vi "LED (SubVI).vi"(8 "error in (no error)":errorcluster, 11 "LED":i8) -> (0 "error out":errorcluster)   [LabVIEW 2017]
uses:
  <vilib>/myRIO/Instrument Drivers/Onboard IO/DIO/typedefs/DIO Reference.ctl
  <vilib>/myRIO/Common/Instrument Driver Framework/Utilities/typedefs/myRIO Generic Hardware Reference.ctl
  <vilib>/myRIO/Common/Instrument Driver Framework/Utilities/typedefs/Hardware Version Enum.ctl
  <vilib>/myRIO/Common/Instrument Driver Framework/Utilities/typedefs/myRIO v1.0 Reference.ctl
  <vilib>/myRIO/Common/Instrument Driver Framework/Utilities/typedefs/Generic FPGA Reference.ctl
  <vilib>/myRIO/Common/Instrument Driver Framework/myRIO v1.0/DIO/typedefs/DIO Channels List.ctl
  <vilib>/myRIO/Common/Instrument Driver Framework/myRIO v1.0/DIO/typedefs/DIO Channels Enum.ctl
  <vilib>/userdefined/High Color/nirio_resource_hc.ctl
  <vilib>/myRIO/Common/Instrument Driver Framework/Utilities/vis/Is FPGA Ref Available.vi
  <vilib>/myRIO/Common/Instrument Driver Framework/myRIO v1.0/DIO/vis/myRIO v1.1 Open DIO.vi
  <vilib>/myRIO/Instrument Drivers/Onboard IO/DIO/vis/Write.vi
  <vilib>/myRIO/Common/Instrument Driver Framework/Utilities/vis/Validate Channels.vi
  <vilib>/myRIO/Common/Instrument Driver Framework/myRIO v1.0/DIO/vis/myRIO v1.0 Reserve DIO.vi
  <vilib>/myRIO/Common/Instrument Driver Framework/myRIO v1.0/Resource Manager/vis/myRIO v1.0 Reserve Channel List.vi
  <vilib>/myRIO/Common/Instrument Driver Framework/myRIO v1.0/DIO/vis/myRIO v1.0 Build MUX Configuration DIO.vi
  <vilib>/myRIO/Common/Instrument Driver Framework/myRIO v1.0/Resource Manager/vis/myRIO v1.0 Reserve Channel.vi
  <vilib>/myRIO/Common/Instrument Driver Framework/myRIO v1.0/Resource Manager/vis/myRIO v1.0 Unreserve Channel.vi
  <vilib>/myRIO/Common/Instrument Driver Framework/myRIO v1.0/Resource Manager/vis/myRIO v1.0 Create Configuration List.vi
  <vilib>/myRIO/Common/Instrument Driver Framework/myRIO v1.0/Resource Manager/vis/myRIO v1.0 Build Mutex Name.vi
  <vilib>/Utility/VariantDataType/GetNumericInfo.vi
  <vilib>/Utility/error.llb/Error Cluster From Error Code.vi
  <vilib>/myRIO/Common/Instrument Driver Framework/myRIO v1.0/myRIO v1.1 Open.vi
  <vilib>/myRIO/Common/Instrument Driver Framework/Utilities/vis/IO Manager.vi
  <vilib>/myRIO/Common/Instrument Driver Framework/Utilities/vis/Configuration Manager.vi
  <vilib>/myRIO/Common/Instrument Driver Framework/myRIO v1.0/Resource Manager/vis/myRIO v1.0 Configure IO.vi
  <vilib>/myRIO/Common/Instrument Driver Framework/myRIO v1.0/myRIO v1.0 Close.vi
  <vilib>/myRIO/Common/Instrument Driver Framework/myRIO v1.0/DIO/vis/myRIO v1.0 Write DIO.vi
  <vilib>/myRIO/Express VI/Onboard IO/DO/DO Express VI.xnode
  <vilib>/myRIO/Instrument Drivers/Onboard IO/DIO/vis/myRIO DIO Open.xnode
  <vilib>/myRIO/Instrument Drivers/Onboard IO/DIO/DIO.lvlib
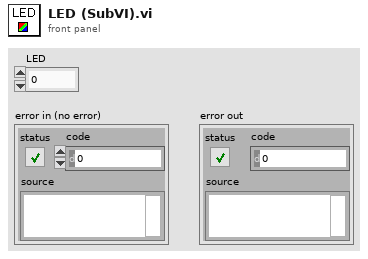
[diagram p1: front panel]
types:
  T1 = typedef "DIO.lvlib/DIO Reference.ctl" = cluster{"myRIO Reference":T2, "DIO Channels List":T6}
  T2 = typedef "myRIO Generic Hardware Reference.ctl" = cluster{"myRIO Model":T3, "myRIO Hardware Reference":T4}
  T3 = typedef "Hardware Version Enum.ctl" = enum16{"Unknown", "myRIO-1900", "myRIO-1950", "roboRIO", "NI ELVIS RIO CM"}
  T4 = typedef "myRIO v1.0 Reference.ctl" = cluster{"Generic FPGA Reference":T5, "Allow multiple opens":bool}
  T5 = typedef "Generic FPGA Reference.ctl" = refnum<k20>
  T6 = typedef "DIO Channels List.ctl" = T7[]
  T7 = typedef "DIO Channels Enum.ctl" = enum16{"Not Connected", "C/DIO0", "C/DIO1", "C/DIO2", "C/DIO3", "C/DIO4", "C/DIO5", "C/DIO6", "C/DIO7", "A/DIO0", "A/DIO1", "A/DIO2", "A/DIO3", "A/DIO4", "A/DIO5", "A/DIO6", "A/DIO7", "A/DIO8", "A/DIO9", "A/DIO10", "A/DIO11", "A/DIO12", "A/DIO13", "A/DIO14", "A/DIO15", "B/DIO0", "B/DIO1", "B/DIO2", "B/DIO3", "B/DIO4", "B/DIO5", "B/DIO6", "B/DIO7", "B/DIO8", "B/DIO9", "B/DIO10", "B/DIO11", "B/DIO12", "B/DIO13", "B/DIO14", "B/DIO15", "LED0", "LED1", "LED2", "LED3", "Button0", "DIO/DIO0", "DIO/DIO1", "DIO/DIO2", "DIO/DIO3", "DIO/DIO4", "DIO/DIO5", "DIO/DIO6", "DIO/DIO7", "DIO/DIO8", "DIO/DIO9", "SPI/CS0", "SPI/CS1", "SPI/CS2", "SPI/CS3", "LED RADIO (Green)", "LED RADIO (Red)", "LED COMM (Green)", "LED COMM (Red)", "LED MODE (Green)", "LED MODE (Red)"}
  T8 = typedef "nirio_resource_hc.ctl" = tag
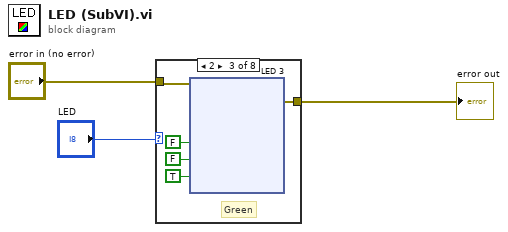
[diagram p0: block diagram]
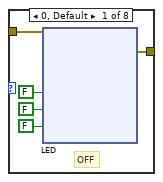
[diagram p2: hidden frame]
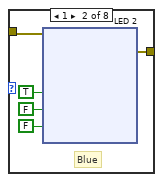
[diagram p3: hidden frame]
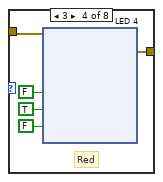
[diagram p4: hidden frame]
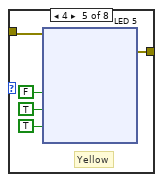
[diagram p5: hidden frame]
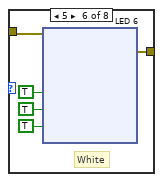
[diagram p6: hidden frame]
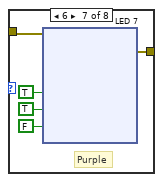
[diagram p7: hidden frame]
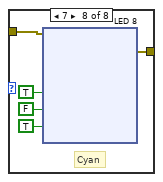
[diagram p8: hidden frame]
diagram:
  n1 = case shown="2" "LED" {
    tunnel: "error in (no error)" -> [w5 w47 w88 w130 w172 w214 w256 w299]
    tunnel: [w4 w46 w89 w131 w173 w215 w257 w298] -> w2
    frame 0, Default {
      # "OFF"
      n2 = xnode "LED"("Blue (A/DIO3 (Pin 17))"=FALSE, "Red (A/DIO4 (Pin 19))"=FALSE, "Green (A/DIO5 (Pin 21))"=FALSE, "error in (no error)"=w5) -> ("error out"=w4:errorcluster)
    }
    frame 1 {
      # "Blue"
      n3 = xnode "LED 2"("Blue (A/DIO3 (Pin 17))"=TRUE, "Red (A/DIO4 (Pin 19))"=FALSE, "Green (A/DIO5 (Pin 21))"=FALSE, "error in (no error)"=w47) -> ("error out"=w46:errorcluster)
    }
    frame 2 {
      # "Green"
      n4 = xnode "LED 3"("Blue (A/DIO3 (Pin 17))"=FALSE, "Red (A/DIO4 (Pin 19))"=FALSE, "Green (A/DIO5 (Pin 21))"=TRUE, "error in (no error)"=w88) -> ("error out"=w89:errorcluster)
    }
    frame 3 {
      # "Red"
      n5 = xnode "LED 4"("Blue (A/DIO3 (Pin 17))"=FALSE, "Red (A/DIO4 (Pin 19))"=TRUE, "Green (A/DIO5 (Pin 21))"=FALSE, "error in (no error)"=w130) -> ("error out"=w131:errorcluster)
    }
    frame 4 {
      # "Yellow"
      n6 = xnode "LED 5"("Blue (A/DIO3 (Pin 17))"=FALSE, "Red (A/DIO4 (Pin 19))"=TRUE, "Green (A/DIO5 (Pin 21))"=TRUE, "error in (no error)"=w172) -> ("error out"=w173:errorcluster)
    }
    frame 5 {
      # "White"
      n7 = xnode "LED 6"("Blue (A/DIO3 (Pin 17))"=TRUE, "Red (A/DIO4 (Pin 19))"=TRUE, "Green (A/DIO5 (Pin 21))"=TRUE, "error in (no error)"=w214) -> ("error out"=w215:errorcluster)
    }
    frame 6 {
      # "Purple"
      n8 = xnode "LED 7"("Blue (A/DIO3 (Pin 17))"=TRUE, "Red (A/DIO4 (Pin 19))"=TRUE, "Green (A/DIO5 (Pin 21))"=FALSE, "error in (no error)"=w256) -> ("error out"=w257:errorcluster)
    }
    frame 7 {
      # "Cyan"
      n9 = xnode "LED 8"("Blue (A/DIO3 (Pin 17))"=TRUE, "Red (A/DIO4 (Pin 19))"=FALSE, "Green (A/DIO5 (Pin 21))"=TRUE, "error in (no error)"=w299) -> ("error out"=w298:errorcluster)
    }
  }
  "error out" <- w2
